vi "Numbers.vi"(0 "Numeric 4":i32=44, 1 "Numeric 5":i16=55, 2 "Numeric 6":i8=66, 3 "Numeric 7":u32=77, 4 "Numeric 8":u16=88, 5 "Numeric 9":u8=99, 6 "Numeric 3":sgl=33.0, 7 "Numeric 10":cxt=11.0+22.0i, 8 "Numeric 2":dbl=22.0, 9 "Numeric 11":cdb=33.0+44.0i, 10 "Numeric":ext=11.0, 11 "Numeric 12":csg=55.0+66.0i, 13 "Numeric 13":i64, 18 "Numeric 15":fxp<+/-,64,32>, 19 "Numeric 14":u64) -> ()   [LabVIEW 2009]
panel:
  in  "stop":bool
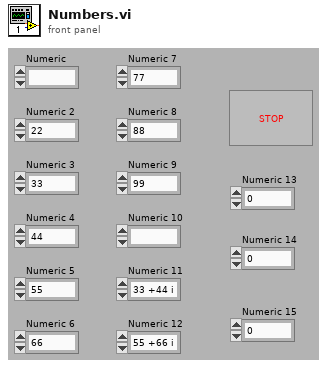
[diagram p1: front panel]
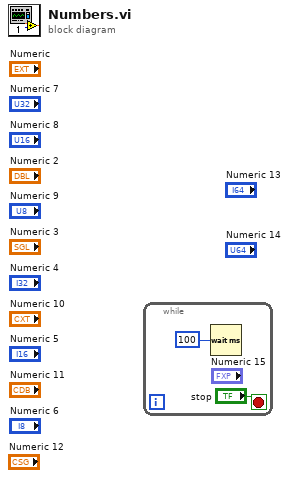
[diagram p0: block diagram]
diagram:
  n1 = while {
    stop <- "stop" stop-if-true
    n2 = Wait (ms)(milliseconds to wait=u32 100) -> ()  [unwired: 1 out]
  }
